vi "Find Workspace.vi"(8 "Error In":errorcluster, 10 "Control In":T2={"I-O.lvclass"=refnum, "Motion.lvclass"=refnum, "Dispenser.lvclass"=refnum}, 11 "Carrier Tray in":refnum<class "Assembly Tray.lvclass">) -> (0 "Error Out":errorcluster, 1 "Workspace":T1, 2 "Control Out":T2, 3 "Carrier Tray Out":refnum<class "Assembly Tray.lvclass">)   [LabVIEW 2016, in "Assembly Tray.lvclass"]
uses:
  Assembly Tray.lvclass
  D:/UCSB-Gantry/V5/Classes/Workspace/Fixture.lvclass
  Controller/Controllers.ctl
  Controller/I-O/I-O.lvclass
  Controller/Motion/A3200/A3200.lvclass
  Controller/Dispenser/Dispenser.lvclass
  Controller/Motion/Motion.lvclass
  Workspace.ctl
  Fixture.lvclass/Fixture.ctl
  Assembly Tray.lvclass/Assembly Tray.ctl
  Read Fixture ID.vi
  Fixture.lvclass
  Controller/Controller.lvclass
panel:
  in  "output cluster 2":T1
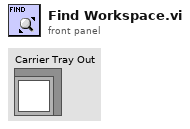
[diagram p1: front panel]
types:
  T1 = typedef "Fixture.lvclass/Workspace.ctl" = cluster{"XYZTheta":dbl[], "Workspace Valve":i32, "Workspace Sensor":i32}
  T2 = typedef "Controller.lvclass/Controllers.ctl" = cluster{"I-O.lvclass":refnum<class "I-O.lvclass">, "Motion.lvclass":refnum<class "Motion.lvclass">, "Dispenser.lvclass":refnum<class "Dispenser.lvclass">}
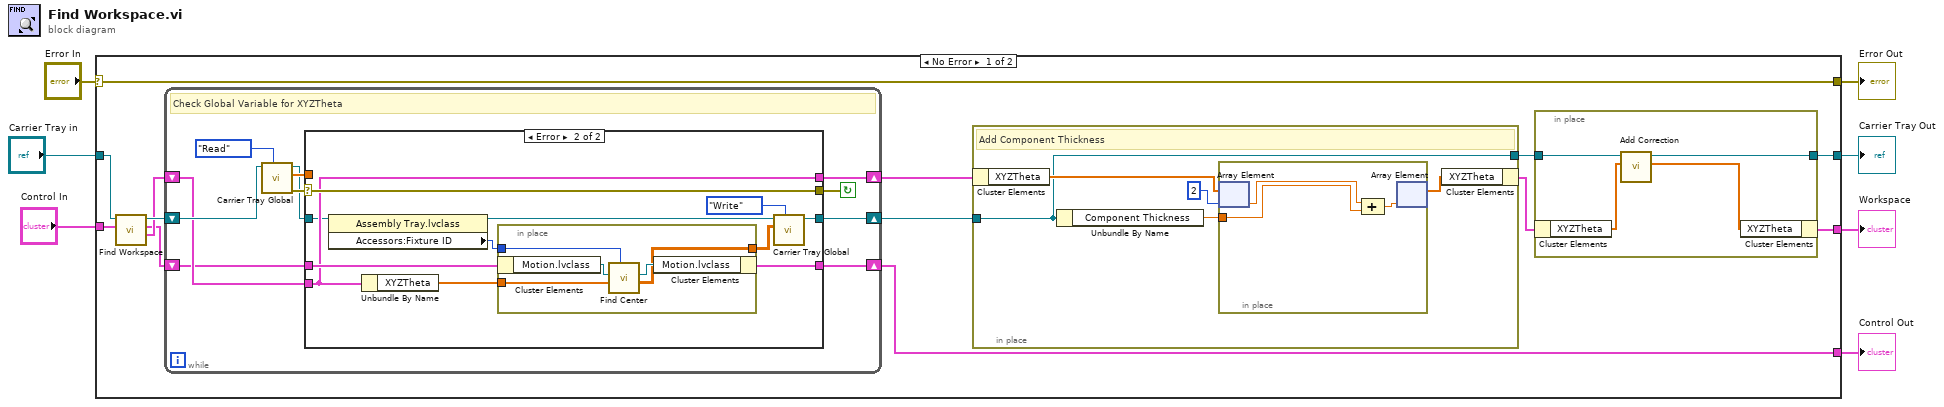
[diagram p0: block diagram]
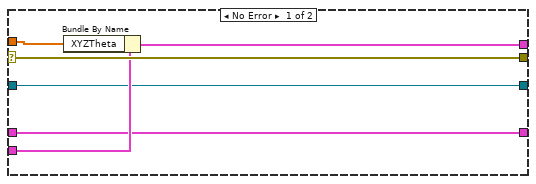
[diagram p2: hidden frame]
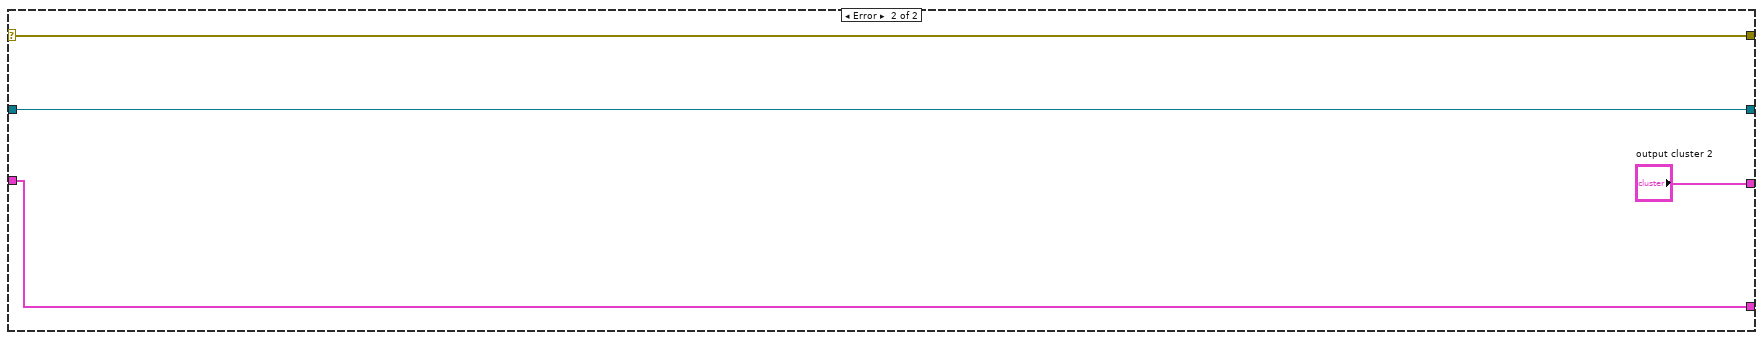
[diagram p3: hidden frame]
diagram:
  n1 = case shown="No Error" "Error In" {
    selector: "Error In" -> [w20 w68]
    tunnel: [w20 w68] -> w6
    tunnel: "Control In" -> [w19 w69]
    tunnel: [w15 w69] -> w4
    tunnel: "Carrier Tray in" -> [w18 w66]
    tunnel: [w16 "output cluster 2"] -> w2
    tunnel: [w17 w66] -> w1
    frame No Error {
      n2 = call-parent "Find Workspace.vi"("Control In"=w19, "Workspace In"=w18) -> (1:"Workspace Out"=w13:T1, "Control Out"=w12:T2, 3:"Workspace Out"=w14:refnum<class "Assembly Tray.lvclass">)  [unwired: 6 in, 1 out]
      n3 = while {
        shift-right: [w34] -> w11
        shift-left: w14 -> [w42]
        shift-right: [w36] -> w15
        shift-left: w12 -> [w37]
        shift-right: [w33] -> w10
        shift-left: w13 -> [w38]
        stop <- w40 continue-if-true
        # "Check Global Variable for XYZTheta"
        n4 = call "Carrier Tray Global.vi"("Action"=enum16{"Initialize", "Read", "Write"}."Read", "Carrier Tray.lvclass"=w42) -> ("error out"=w41:errorcluster, "XYZTheta out"=w39:dbl[], "Carrier Tray.lvclass 2"=w35:refnum<class "Assembly Tray.lvclass">)  [unwired: 7 in]
        n5 = case shown="Error" w41 {
          selector: w41 -> [w49 w60]
          tunnel: [w49 w60] -> w40
          tunnel: w39 -> [w48 _]
          tunnel: [w47 w54] -> w33
          tunnel: w38 -> [w46 w54]
          tunnel: w37 -> [w44 w59]
          tunnel: [w44 w58] -> w36
          tunnel: w35 -> [w45 w52]
          tunnel: [w45 w57] -> w34
          frame No Error {
            n6 = Bundle By Name(cluster=w46, "XYZTheta"=w48) -> (w47:T1)
          }
          frame Error {
            n7 = property class="Assembly Tray.lvclass"(reference=w52) -> (reference out=w51:refnum<class "Assembly Tray.lvclass">, "Accessors:Fixture ID"=w50:i32)  [unwired: 1 in, 1 out]
            n8 = Unbundle By Name(w54) -> ("XYZTheta"=w53:dbl[])
            n9 = in-place {
              in-place-border: [w63] -> w55
              in-place-border: w53 -> [w62]
              in-place-border: w50 -> [w61]
              n10 = in-place-cluster #1(w59) -> ("Motion.lvclass"=w64:refnum<class "Motion.lvclass">)
              n11 = call "Find Center.vi"("Tray Number"=w61, "XYZTheta"=w62, "Motion.lvclass"=w64) -> ("XYZTheta Centers"=w63:dbl[][], "Motion Out"=w65:refnum<class "Motion.lvclass">)  [unwired: 7 in]
              n12 = in-place-cluster #1("Motion.lvclass"=w65) -> (w58:T2)
            }
            n13 = call "Carrier Tray Global.vi"("Action"=enum16{"Initialize", "Read", "Write"}."Write", "XYZTheta in"=w55, "Carrier Tray.lvclass"=w51) -> ("Carrier Tray.lvclass 2"=w57:refnum<class "Assembly Tray.lvclass">)  [unwired: 6 in, 2 out]
          }
        }
      }
      n14 = in-place {
        in-place-border: w11 -> [w21]
        in-place-border: [w21] -> w9
        # "Add Component Thickness"
        n15 = in-place-cluster #2(w10) -> ("XYZTheta"=w24:dbl[])
        n16 = Unbundle By Name(w21) -> ("Component Thickness"=w22:dbl)
        n17 = in-place {
          in-place-border: w22 -> [w27]
          n18 = in-place-array #3(w24, 2) -> (w28:dbl)
          n19 = Compound Arithmetic op=ADD(w28, w27) -> (w26:dbl)
          n20 = in-place-array #3(w26) -> (w23:dbl[])  [unwired: 1 out]
        }
        n21 = in-place-cluster #2("XYZTheta"=w23) -> (w8:T1)
      }
      n22 = in-place {
        in-place-border: [w32] -> w17
        in-place-border: w9 -> [w31]
        n23 = in-place-cluster #4(w8) -> ("XYZTheta"=w30:dbl[])
        n24 = call "Add Correction.vi"("XYZTheta"=w30, "Carrier Tray in"=w31) -> ("XYZTheta Out"=w29:dbl[], "Carrier Tray out"=w32:refnum<class "Assembly Tray.lvclass">)  [unwired: 7 in, 1 out]
        n25 = in-place-cluster #4("XYZTheta"=w29) -> (w16:T1)
      }
    }
    frame Error {
    }
  }
  "Error Out" <- w6
  "Control Out" <- w4
  "Workspace" <- w2
  "Carrier Tray Out" <- w1
